vi "Configure Device.vi"(8 "error in":errorcluster, 11 "DAQ HVPS in":refnum<class "DAQ HVPS.lvclass">) -> (0 "error out":errorcluster, 3 "DAQ HVPS out":refnum<class "DAQ HVPS.lvclass">)   [LabVIEW 2013, in "DAQ HVPS.lvclass"]
doc: "Get the information from the configuration file regarding the operation fo the DAQ based HVPS. The information is:\n\n* <b>DAQ.AI</b> - string defining the physical channel for the analog input\n* <b>DAQ.AO</b> - string defining the physical channel for the analog output\n* <b>DAQ.Enable</b> - physical channel for the Enable signal\n* <b>DAQ.Scale</b> - numeric defining the conversion of DAQ voltage to a power supply voltage\n* <b>V0</b> - numeric defining the startup setting for the voltage\n* <b>DAQ.On?</b> - boolean defining the initial operational state of the device\n\nUpon successful completion of retrieval from the configuration file, close the session to the config file."
uses:
  DAQ HVPS.lvclass
  Configurable Device/Configurable Device.lvclass/Configurable Device.ctl
  Reusable/Session APIs/File Access/Config Data/Config Data.lvclass/Config Data.ctl
  Reusable/Session APIs/File Access/Config Data/Accessors/Read Ref.vi
  Configurable Device/Read Handle.vi
  <vilib>/Utility/config.llb/Read Key (String).vi
  <vilib>/Utility/config.llb/Read Key (Double).vi
  <vilib>/Utility/config.llb/Read Key (Boolean).vi
  Configure AI.vi
  Configure AO.vi
  Configure DO.vi
  Reusable/Session APIs/File Access/Config Data/Config Data.lvclass
  <vilib>/Utility/config.llb/NI_LVConfig.lvlib
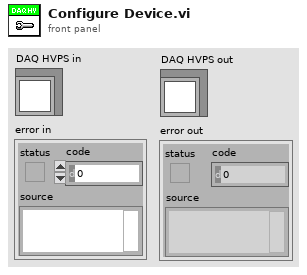
[diagram p1: front panel]
types:
  T1 = typedef "Config Data.lvclass/Config Session.ctl" = refnum<data-value>
  T2 = typedef "NI_LVConfig.lvlib/Config Data RefNum.ctl" = refnum<k1>
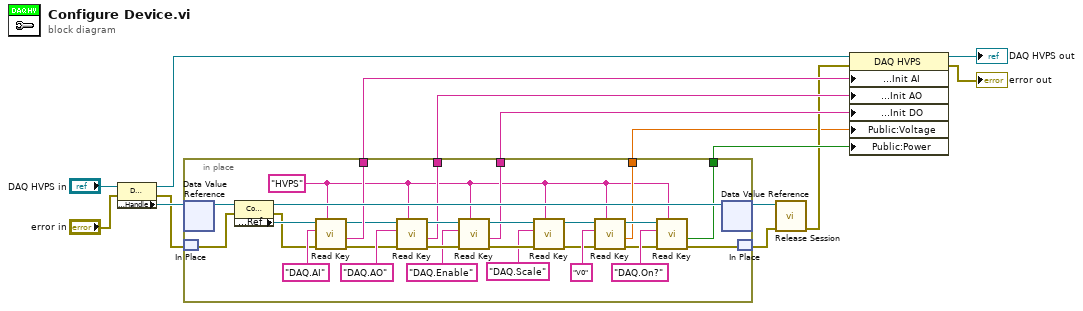
[diagram p0: block diagram]
diagram:
  n1 = property class="DAQ HVPS"(reference="DAQ HVPS in", error in="error in") -> (reference out=w7:refnum<class "DAQ HVPS.lvclass">, error out=w14:errorcluster, "Accessors:Handle"=w15:T1)
  n2 = in-place {
    in-place-border: [w31] -> w8
    in-place-border: [w30] -> w5
    in-place-border: [w29] -> w6
    in-place-border: [w28] -> w4
    in-place-border: [w17] -> w2
    w16 = "HVPS" ("section")
    n3 = in-place-dvr #1(w15) -> (w43:refnum<class "Config Data.lvclass">)  [unwired: 1 out]
    n4 = in-place-match #2(w14) -> (w27:errorcluster)
    n5 = property class="Config Data"(reference=w43, error in=w27) -> (reference out=w40:refnum<class "Config Data.lvclass">, error out=w26:errorcluster, "Accessors:Ref"=w42:T2)
    n6 = call-poly <vilib>:"Read Key.vi"("section"=w16, "error in (no error)"=w26, "key"="DAQ.AI" ("section"), "refnum"=w42) -> ("error out"=w23:errorcluster, "value"=w30:string, "refnum out"=w24:T2)  [unwired: 4 in, 1 out]
    n7 = call-poly <vilib>:"Read Key.vi"("section"=w16, "error in (no error)"=w23, "key"="DAQ.AO", "refnum"=w24) -> ("error out"=w37:errorcluster, "value"=w29:string, "refnum out"=w38:T2)  [unwired: 4 in, 1 out]
    n8 = call-poly <vilib>:"Read Key.vi"("section"=w16, "error in (no error)"=w37, "key"="DAQ.Enable", "refnum"=w38) -> ("error out"=w34:errorcluster, "value"=w28:string, "refnum out"=w35:T2)  [unwired: 4 in, 1 out]
    n9 = call-poly <vilib>:"Read Key.vi"("section"=w16, "error in (no error)"=w34, "key"="DAQ.Scale", "refnum"=w35) -> ("error out"=w20:errorcluster, "refnum out"=w21:T2)  [unwired: 4 in, 2 out]
    n10 = call-poly <vilib>:"Read Key.vi"("section"=w16, "error in (no error)"=w20, "key"="V0", "refnum"=w21) -> ("error out"=w18:errorcluster, "value"=w17:dbl, "refnum out"=w19:T2)  [unwired: 4 in, 1 out]
    n11 = call-poly <vilib>:"Read Key.vi"("section"=w16, "error in (no error)"=w18, "key"="DAQ.On?", "refnum"=w19) -> ("error out"=w25:errorcluster, "value"=w31:bool)  [unwired: 4 in, 2 out]
    n12 = in-place-dvr #1(w40) -> (w13:T1)  [unwired: 1 out]
    n13 = in-place-match #2(w25) -> (w12:errorcluster)
  }
  n14 = call "Release Session.vi"("error in"=w12, "Session Handle"=w13) -> ("error out"=w3:errorcluster)  [unwired: 8 in, 1 out]
  n15 = property class="DAQ HVPS"(reference=w7, error in=w3, "Hardware Configuration:Init AI"=w5, "Hardware Configuration:Init AO"=w6, "Hardware Configuration:Init DO"=w4, "Public:Voltage"=w2, "Public:Power"=w8) -> (reference out=→"DAQ HVPS out":refnum<class "DAQ HVPS.lvclass">, error out=→"error out":errorcluster)
